vi "_MDPtr ForceDeletePtr.vi"(9 "error in (no error)":errorcluster, 10 "HexStrPtr":T1) -> (2 "error out":errorcluster, 3 "HexStrPtr (dup)":T1)   [LabVIEW 2014]
uses:
  MDPtr TypeDef/MDPtr.ctl
  MDPtr TypeDef/MDPtr DataFrame-PlaceHolder.ctl
  MDPtr TypeDef/MDPtr DataFrame-Common.ctl
  MDPtr TypeDef/MDPtr SupportedDataTypeDef.ctl
  _MDPtr Build Error Cluster.vi
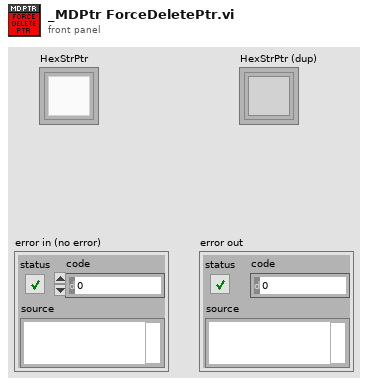
[diagram p1: front panel]
types:
  T1 = typedef "MDPtr.ctl" = refnum<k1>
  T2 = typedef "MDPtr DataFrame-PlaceHolder.ctl" = cluster{"Common":T3, "DVR":refnum<data-value>}
  T3 = typedef "MDPtr DataFrame-Common.ctl" = cluster{"Data Type":T4, "Copy Count":i32, "String Attribute":string}
  T4 = typedef "MDPtr SupportedDataTypeDef.ctl" = enum16{"<Invalid>", "Waveform", "Waveform Arr", "Double Arr", "String Arr"}
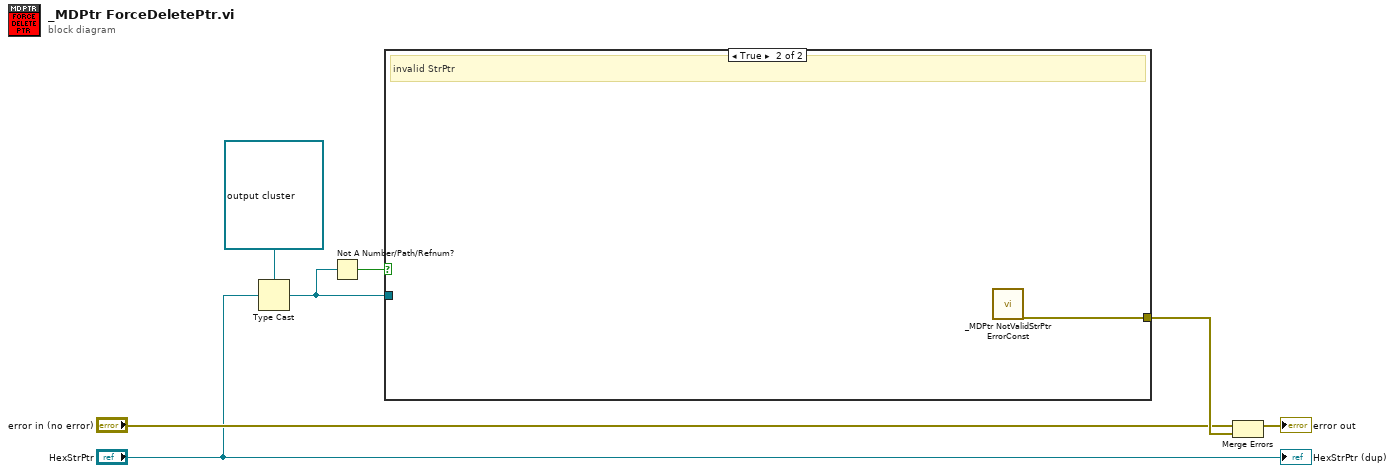
[diagram p0: block diagram]
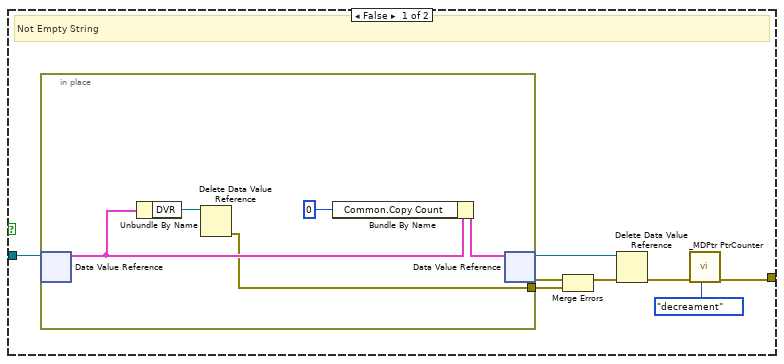
[diagram p2: hidden frame]
diagram:
  n1 = Type Cast(type=refnum<data-value> refnum ("data value reference"), x="HexStrPtr") -> (*(type *) &x=w1:refnum<data-value>)
  n2 = Not A Number/Path/Refnum?(number/path/refnum=w1) -> (NaN/Path/Refnum?=w2:bool)
  n3 = case shown="True" w2 {
    tunnel: [w9 w21] -> w7
    tunnel: w1 -> [w14 _]
    frame False {
      # "Not Empty String"
      n4 = in-place {
        in-place-border: [w16] -> w10
        n5 = in-place-dvr #1(w14) -> (w20:T2)  [unwired: 1 out]
        n6 = Unbundle By Name(w20) -> ("DVR"=w17:refnum<data-value>)
        n7 = Delete Data Value Reference(data value reference=w17) -> (error out=w16:errorcluster)  [unwired: 1 in, 1 out]
        n8 = Bundle By Name(cluster=w20, "Common.Copy Count"=0) -> (w19:T2)
        n9 = in-place-dvr #1(w19) -> (w12:refnum<data-value>, w15:errorcluster)
      }
      n10 = Merge Errors(w15, w10) -> (w11:errorcluster)
      n11 = Delete Data Value Reference(data value reference=w12, error in=w11) -> (error out=w13:errorcluster)  [unwired: 1 out]
      n12 = call "_MDPtr PtrCounter.vi"("Oper(Get)"=enum16{"GET", "Increament", "decreament"}."decreament", "error in (no error)"=w13) -> ("error out"=w9:errorcluster)  [unwired: 8 in, 1 out]
    }
    frame True {
      # "invalid StrPtr"
      n13 = call "_MDPtr NotValidStrPtr ErrorConst.vi"() -> ("error out"=w21:errorcluster)  [unwired: 19 in]
    }
  }
  n14 = Merge Errors("error in (no error)", w7) -> (→"error out":errorcluster)
  "HexStrPtr (dup)" <- "HexStrPtr"
